vi "matrici_v0_v21.vi"() -> ()   [LabVIEW 2009]
panel:
  in  "h":dbl(slide)=127.46113989637304 scale=0.0..400.0
  in  "d":dbl(knob)=7.878743086825296 scale=0.0..10.0
  in  "v":dbl(slide)=93.03135888501741 scale=300.0..0.0
  out "Iteratia":dbl=54.0
  in  "stop":bool
  out "Picture":picture
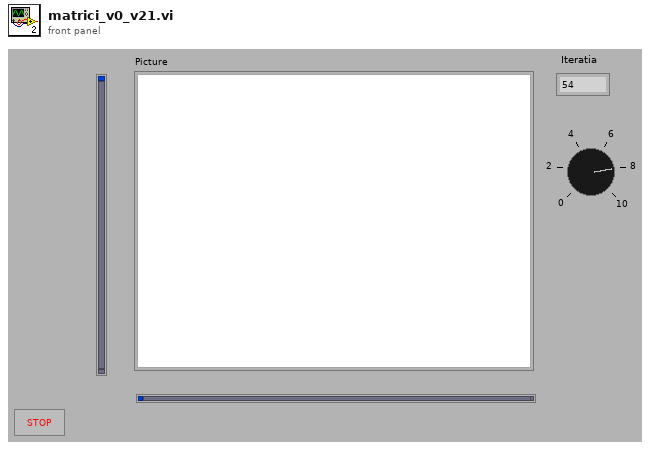
[diagram p1: front panel]
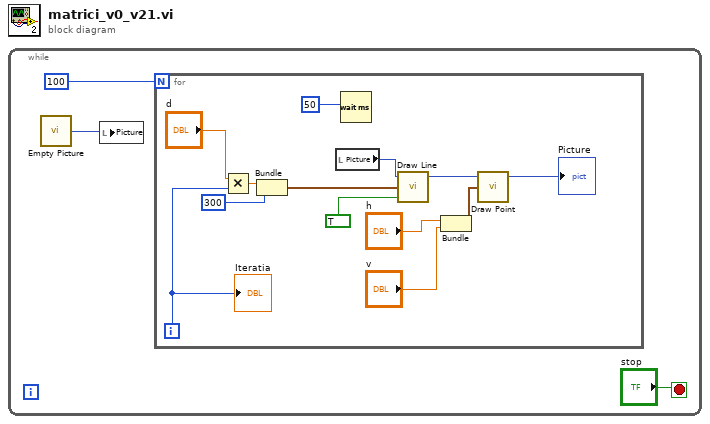
[diagram p0: block diagram]
diagram:
  n1 = while {
    stop <- "stop" stop-if-true
    n2 = call "Empty Picture"() -> ("empty picture"=w1:picture)
    n3 = local write "Picture"(w1) -> ()
    n4 = for {
      N: 100 -> [_]
      i -> [w9]
      n5 = Multiply(x="d", y=w9) -> (x*y=w7:dbl)
      n6 = Bundle(w7, 300) -> (w14:cluster{dbl, i32})  [unwired: 1 in]
      n7 = local read "Picture"() -> (w16:picture)
      n8 = Wait (ms)(milliseconds to wait=50) -> ()  [unwired: 1 out]
      n9 = call <vilib>:"Draw Line.vi"("picture"=w16, "end point"=w14, "absolute coordinates?(T)"=TRUE) -> ("new picture"=w15:picture)  [unwired: 6 in]
      n10 = Bundle("h"="h", "v"="v") -> (w10:cluster{"h":dbl, "v":dbl})  [unwired: 1 in]
      n11 = call <vilib>:"Draw Point.vi"("picture"=w15, "point(x,y)"=w10) -> ("new picture"=→"Picture":picture)  [unwired: 7 in]
      "Iteratia" <- w9
    }
  }
